vi "Instrument Control Project (FINAL).vi"() -> ()   [LabVIEW 2017]
panel:
  out "Instrument Name":string
  out "Oscilloscope Display":dbl[][](graph)
  out "Vin/Vout":cluster{"Y":dbl[], "Y":dbl[]}[](graph)
  in  "Upper Frequency (kHz)":dbl=1.0 min=0.0 step=0.5
  in  "Lower Frequency (kHz)":dbl=1.0 min=0.0 step=0.5
  # "BEFORE RUNNING:\n1- Turn on signal generator (Tektronix AFG1022) and oscilloscope (Agilent DSO1002A)\n2- Put channel 1 on Vin and channel 2 and Vout\n3- Confirm lowpass filter circuit is correct (1k resistor and 30 nF capacitor) and grounded properly\n4- Open all VI's in Instrument Control Project Folder\n6- Run Instrument ControlProject VI program without frequencies defined, confirm instrument name to be: TEKTR\n7- Select frequencies\n8- Run program\n9- Add comment\n10- Save file\n\n*** If 9.9E37 is returned in dataset or Vout/Vin Graph rerun the program***"
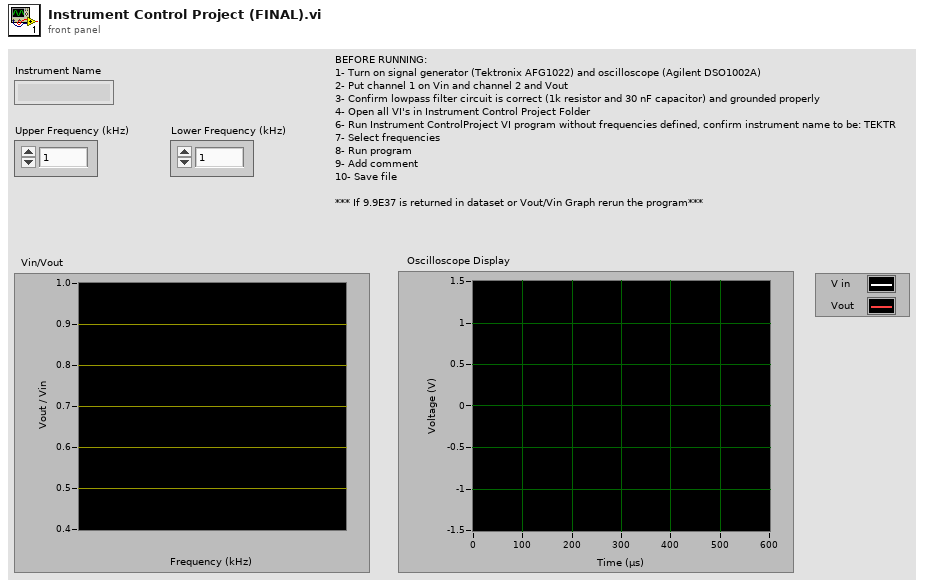
[diagram p1: front panel]
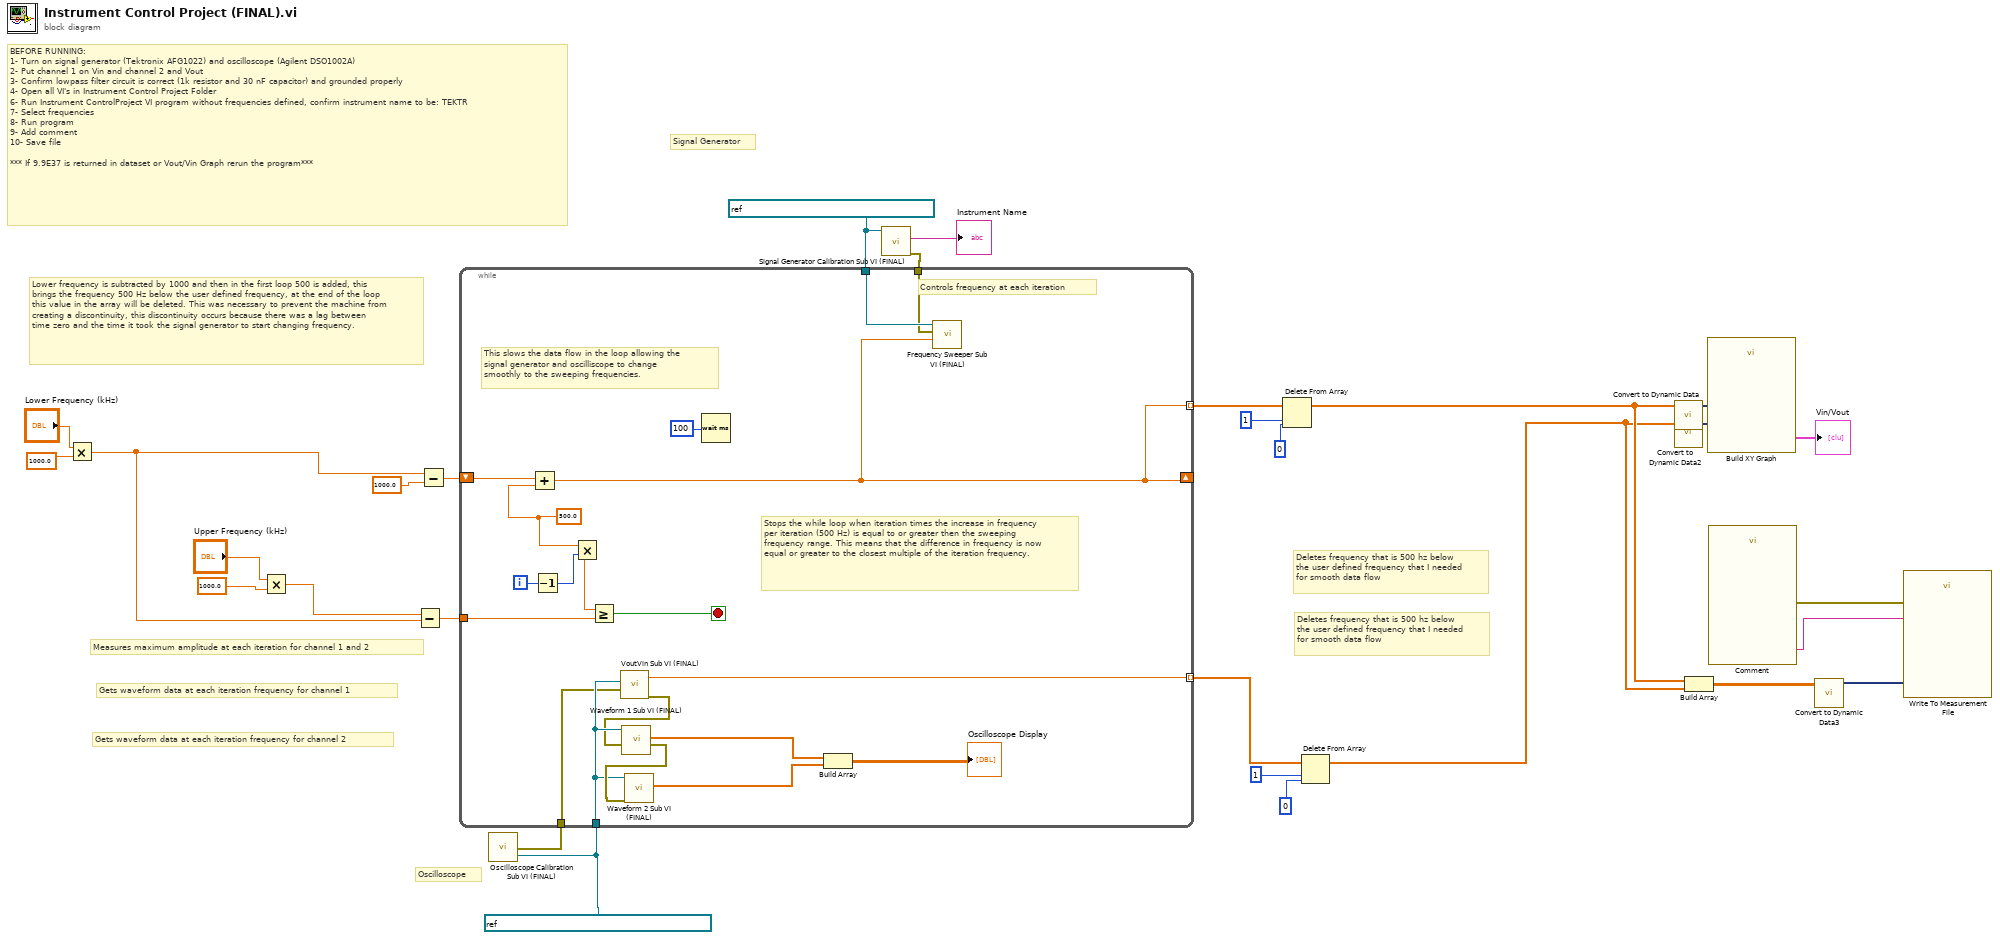
[diagram p0: block diagram]
diagram:
  w7 = refnum<visa-resource-name> "USB0::0x0699::0x0353::1612076::INSTR" ("VISA resource name")
  w2 = refnum<visa-resource-name> "USB0::0x0957::0x0588::CN49221468::INSTR" ("VISA resource name")
  # "Oscilloscope"
  # "Signal Generator"
  # "Deletes frequency that is 500 hz below the user defined frequency that I needed for smooth data flow"
  # "Gets waveform data at each iteration frequency for channel 2"
  # "Gets waveform data at each iteration frequency for channel 1"
  # "Measures maximum amplitude at each iteration for channel 1 and 2"
  # "Deletes frequency that is 500 hz below the user defined frequency that I needed for smooth data flow"
  # "Lower frequency is subtracted by 1000 and then in the first loop 500 is added, this brings the frequency 500 Hz below the user defined frequency, at the end of the loop this value in the array will be deleted. This was necessary to prevent the machine from creating a discontinuity, this discontinuity occurs because there was a lag between time zero and the time it took the signal generator to start changing frequency."
  # "BEFORE RUNNING:\n1- Turn on signal generator (Tektronix AFG1022) and oscilloscope (Agilent DSO1002A)\n2- Put channel 1 on Vin and channel 2 and Vout\n3- Confirm lowpass filter circuit is correct (1k resistor and 30 nF capacitor) and grounded properly\n4- Open all VI's in Instrument Control Project Folder\n6- Run Instrument ControlProject VI program without frequencies defined, confirm instrument name to be: TEKTR\n7- Select frequencies\n8- Run program\n9- Add comment\n10- Save file\n\n*** If 9.9E37 is returned in dataset or Vout/Vin Graph rerun the program***"
  n1 = Multiply(x="Lower Frequency (kHz)", y=1000.0) -> (x*y=w20:dbl)
  n2 = Multiply(x="Upper Frequency (kHz)", y=1000.0) -> (x*y=w28:dbl)
  n3 = Subtract(x=w28, y=w20) -> (x-y=w24:dbl)
  n4 = Subtract(x=w20, y=1000.0) -> (x-y=w19:dbl)
  n5 = call "Oscilloscope Calibration Sub VI (FINAL).vi"("VISA resource name"=w2) -> ("error out"=w1:errorcluster)  [unwired: 1 in]
  n6 = call "Signal Generator Calibration Sub VI (FINAL).vi"("VISA resource name"=w7) -> ("error out"=w6:errorcluster, "Confirmed Instrument Name"=→"Instrument Name":string)  [unwired: 1 in]
  n7 = while {
    shift-right: [w39] -> _
    shift-left: w19 -> [w48]
    tunnel: w24 -> [w45]
    tunnel: [w33] -> w22 mode=indexing
    tunnel: [w39] -> w16 mode=indexing
    tunnel: w2 -> [w35]
    tunnel: w7 -> [w40]
    tunnel: w6 -> [w38]
    tunnel: w1 -> [w32]
    i -> [w31]
    stop <- w47 stop-if-true
    w44 = 500.0 ("y")
    # "This slows the data flow in the loop allowing the signal generator and oscilliscope to change smoothly to the sweeping frequencies."
    # "Controls frequency at each iteration"
    # "Stops the while loop when iteration times the increase in frequency per iteration (500 Hz) is equal to or greater then the sweeping frequency range. This means that the difference in frequency is now equal or greater to the closest multiple of the iteration frequency."
    n8 = Add(x=w48, y=w44) -> (x+y=w39:dbl)
    n9 = Decrement(x=w31) -> (x-1=w30:i32)
    n10 = Multiply(x=w44, y=w30) -> (x*y=w43:dbl)
    n11 = Greater Or Equal?(x=w43, y=w45) -> (x >= y?=w47:bool)
    n12 = call "VoutVin Sub VI (FINAL).vi"("error in (no error)"=w32, "VISA Refnum in"=w35) -> ("error out"=w34:errorcluster, "Numeric"=w33:dbl)
    n13 = call "Waveform 1 Sub VI (FINAL).vi"("error in (no error)"=w34, "VISA Refnum in"=w35) -> ("error out"=w37:errorcluster, "Array"=w42:dbl[])  [unwired: 8 in]
    n14 = call "Waveform 2 Sub VI (FINAL).vi"("error in (no error)"=w37, "VISA Refnum in"=w35) -> ("Array"=w36:dbl[])  [unwired: 1 out]
    n15 = Wait (ms)(milliseconds to wait=u32 100) -> ()  [unwired: 1 out]
    n16 = Build Array(w42, w36) -> (→"Oscilloscope Display":dbl[][])
    n17 = call "Frequency Sweeper Sub VI (FINAL).vi"("Numeric"=w39, "error in (no error)"=w38, "VISA resource name"=w40) -> ()  [unwired: 1 out]
  }
  n18 = Delete From Array(array=w16, length=1, index=0) -> (array with subset deleted=w11:dbl[])  [unwired: 1 out]
  n19 = Delete From Array(array=w22, length=1, index=0) -> (array with subset deleted=w10:dbl[])  [unwired: 1 out]
  n20 = call "Convert to Dynamic Data"("Array"=w11) -> ("Dynamic Data Type"=w15:dynamicdata)  [unwired: 3 in]
  n21 = call "Convert to Dynamic Data2"("Array"=w10) -> ("Dynamic Data Type"=w14:dynamicdata)  [unwired: 3 in]
  n22 = Build Array(w11, w10) -> (w9:dbl[][])
  n23 = call "Build XY Graph"("Y Input"=w14, "X Input"=w15) -> ("XY Graph"=→"Vin/Vout":cluster{"X":dbl[], "Y":dbl[]}[])  [unwired: 8 in, 1 out]
  n24 = call "Comment"() -> ("Comment"=w3:string, "error out"=w4:errorcluster)  [unwired: 17 in, 1 out]
  n25 = call "Convert to Dynamic Data3"("2D Array"=w9) -> ("Dynamic Data Type"=w8:dynamicdata)  [unwired: 3 in]
  n26 = call "Write To Measurement File"("Signals"=w8, "error in (no error)"=w4, "Comment"=w3) -> ()  [unwired: 14 in, 3 out]
